vi "throw not found error.vi"(8 "error in (no error)":errorcluster, 11 "id":string) -> (0 "error out":errorcluster)   [LabVIEW 2017]
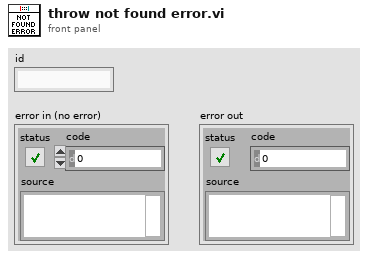
[diagram p1: front panel]
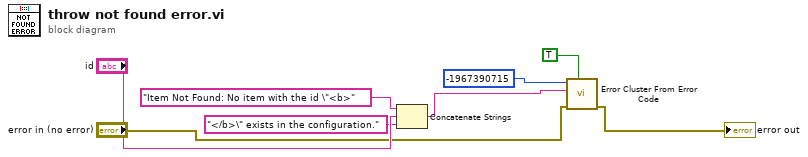
[diagram p0: block diagram]
diagram:
  n1 = Concatenate Strings("Item Not Found: No item with the id \"<b>" ("initial string"), "id", "</b>\" exists in the configuration." ("string")) -> (w4:string)
  n2 = call <vilib>:"Error Cluster From Error Code.vi"("show call chain? (False)"=TRUE, "error in (no error)"="error in (no error)", "error message (\"\")"=w4, "error code (0)"=-1967390715) -> ("error out"=→"error out":errorcluster)  [unwired: 5 in]
